vi "ROS_UDP Server.vi"(2 "IP":string, 3 "Occurrence in":refnum<k4>) -> ()   [LabVIEW 2014]
doc: "Opens a UDP server, writes to the server, and then closes the connection"
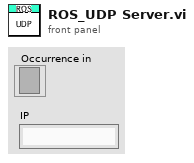
[diagram p1: front panel]
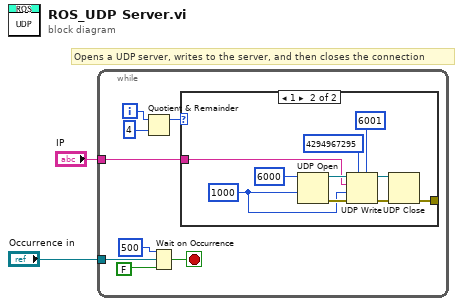
[diagram p0: block diagram]
diagram:
  # "Opens a UDP server, writes to the server, and then closes the connection"
  n1 = while {
    tunnel: "IP" -> [w10]
    tunnel: "Occurrence in" -> [w3]
    i -> [w7]
    stop <- w4 stop-if-true
    n2 = Quotient & Remainder(x=w7, y=4) -> (x-y*floor(x/y)=w9:i32)  [unwired: 1 out]
    n3 = Wait on Occurrence(1:FALSE ("ignore previous (T)"), 2:w3, 3:500 ("ms timeout (-1)")) -> (0:w4:bool)
    n4 = case shown="1" w9 {
      tunnel: w10 -> [_ w13]
      tunnel: [_ w11] -> _
      frame 0, Default {
      }
      frame 1 {
        w12 = 1000 ("timeout ms (25000)")
        n5 = UDP Open(9:w12, 11:u16 6000 ("port")) -> (port=w15:refnum<k16>, 0:w14:errorcluster)  [unwired: 3 in, 1 out]
        n6 = UDP Write(address=u32 4294967295, port or service name=u16 6001, connection ID=w15, data in=w13, 8:w14, 9:w12) -> (error out=w16:errorcluster, 3:w17:refnum<k16>)
        n7 = UDP Close(connection ID=w17, 8:w16) -> (error out=w11:errorcluster)  [unwired: 1 out]
      }
    }
  }
